vi "New VI.vi"(8 "error in":errorcluster) -> (0 "error out":errorcluster, 3 "VI Refnum":refnum<vi>)   [LabVIEW 2026, in "G-AI Core.lvlib"]
doc: "Creates a new VI and returns it's reference. It's a simple wrapper around the New VI VI-Scripting function. Use this over the original function, since it keeps the VI reference alive even if the tools execution has finished.\n\n_____\nCreated using DQMH Framework: Event Scripter 7.1.2.1547."
uses:
  G-AI Core.lvlib
  New VI Argument--cluster.ctl
  New VI (Reply Payload)--cluster.ctl
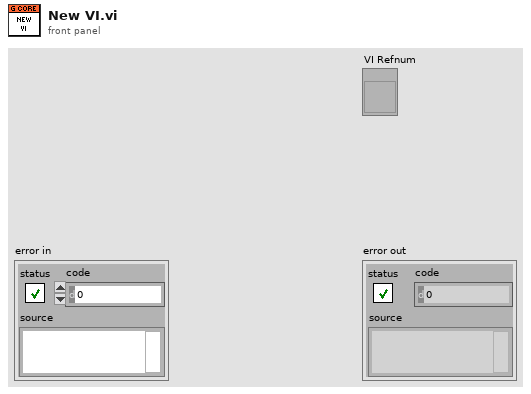
[diagram p1: front panel]
types:
  T1 = typedef "G-AI Core.lvlib/New VI Argument--cluster.ctl" = cluster{"Wait Notifier":refnum<notifier>, "wait for reply":bool}
  T2 = typedef "G-AI Core.lvlib/Request Events--cluster.ctl" = cluster{"Stop Module":refnum<user-event>, "Show Panel":refnum<user-event>, "Hide Panel":refnum<user-event>, "Get Module Execution Status":refnum<user-event>, "Show Diagram":refnum<user-event>, "Store Reference":refnum<user-event>, "Get Reference":refnum<user-event>, "New VI":refnum<user-event>, "Open VI Reference":refnum<user-event>}
  T3 = typedef "G-AI Core.lvlib/New VI (Reply Payload)--cluster.ctl" = cluster{"VI Refnum":refnum<vi>, "error":errorcluster}
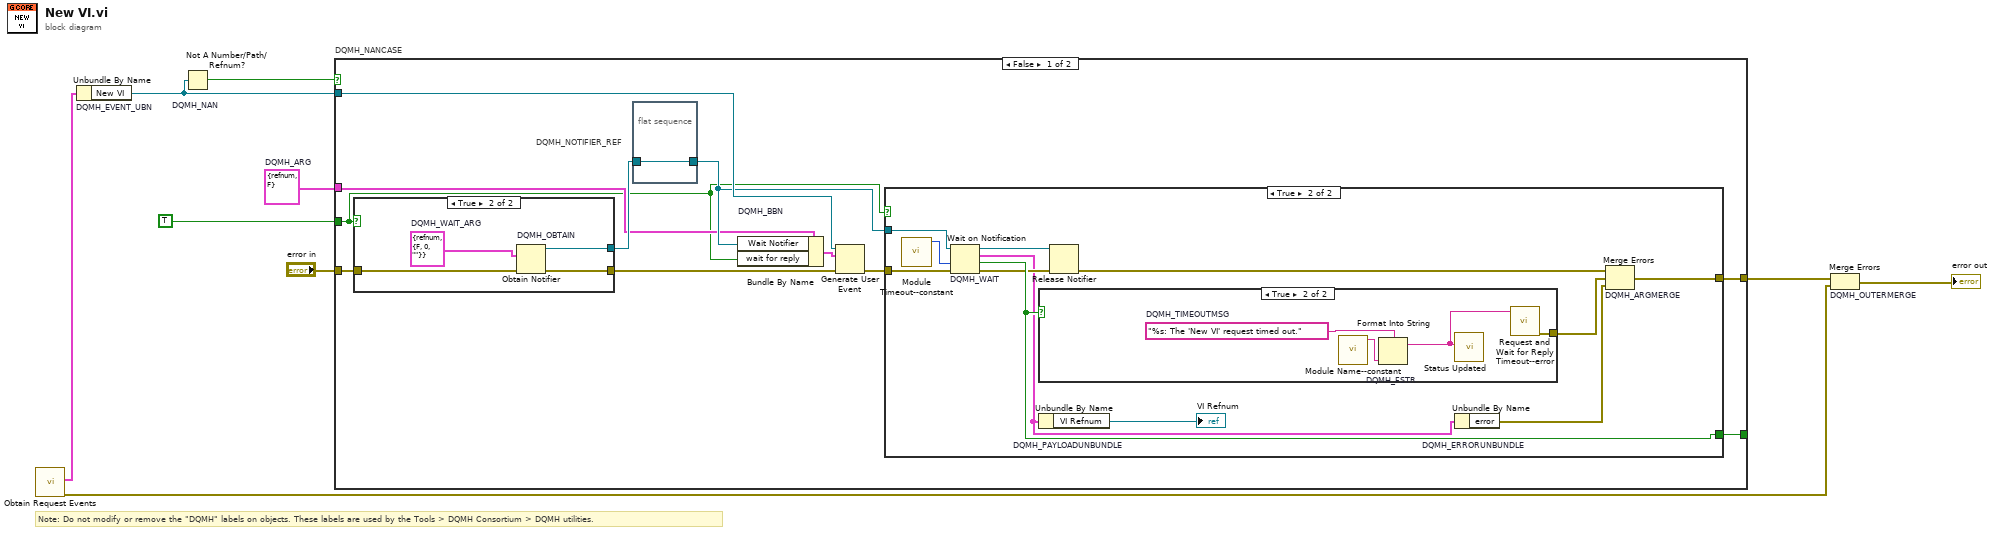
[diagram p0: block diagram]
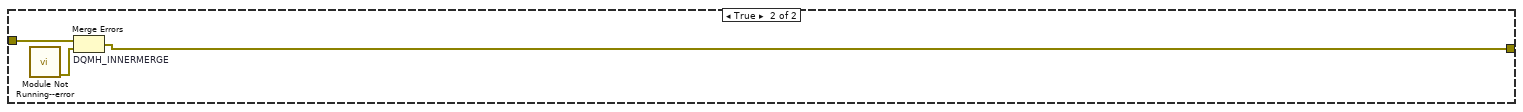
[diagram p5: hidden frame]
diagram:
  w4 = T1 {"Wait Notifier"=refnum, "wait for reply"=FALSE}  # DQMH_ARG
  # "Note: Do not modify or remove the \"DQMH\" labels on objects. These labels are used by the Tools > DQMH Consortium > DQMH utilities."
  n1 = call "Obtain Request Events.vi"() -> ("error out"=w2:errorcluster, "G-AI Core Request Events"=w1:T2)  [unwired: 10 in]
  n2 = Unbundle By Name "DQMH_EVENT_UBN"(w1) -> ("New VI"=w7:refnum<user-event>)
  n3 = Not A Number/Path/Refnum? "DQMH_NAN"(number/path/refnum=w7) -> (NaN/Path/Refnum?=w6:bool)
  n4 = case "DQMH_NANCASE" shown="False" w6 {
    tunnel: "error in" -> [w20 w46]
    tunnel: w7 -> [w18 _]
    tunnel: [w15 w45] -> w5
    tunnel: [w16 _] -> _
    tunnel: w4 -> [w11 _]
    tunnel: TRUE ("wait for reply (T)") -> [w10 _]
    frame False {
      n5 = case shown="True" w10 {
        tunnel: w20 -> [w39 w43]
        tunnel: [w39 w42] -> w17
        tunnel: [_ w40] -> w13
        frame False {
        }
        frame True {
          w41 = T3 {"VI Refnum"=refnum, "error"={"status"=FALSE, "code"=0, "source"=""}}  # DQMH_WAIT_ARG
          n6 = Obtain Notifier "DQMH_OBTAIN"(notification data type=w41, error in (no error)=w43) -> (notifier out=w40:refnum<notifier>, error out=w42:errorcluster)  [unwired: 2 in, 1 out]
        }
      }
      n7 = flat-sequence "DQMH_NOTIFIER_REF" {
        tunnel: w13 -> [w21]
        tunnel: [w21] -> w12
        frame #0 {
        }
      }
      n8 = Bundle By Name "DQMH_BBN"(cluster=w11, "Wait Notifier"=w12, "wait for reply"=w10) -> (w14:T1)
      n9 = Generate User Event(user event=w18, event data cluster=w14, error in=w17) -> (error out=w19:errorcluster)  [unwired: 1 in, 1 out]
      n10 = case shown="True" w10 {
        tunnel: w19 -> [w22 w34]
        tunnel: w12 -> [_ w33]
        tunnel: [_ w31] -> w16
        tunnel: [w22 w30] -> w15
        frame False {
        }
        frame True {
          n11 = call "Module Timeout--constant.vi"() -> ("Module Timeout"=w24:i32)  [unwired: 11 in]
          n12 = Wait on Notification "DQMH_WAIT"(notifier=w33, timeout in ms (-1)=w24, error in (no error)=w34) -> (notifier out=w32:refnum<notifier>, notification=w25:T3, timed out?=w31:bool, error out=w29:errorcluster)  [unwired: 1 in]
          n13 = case shown="True" w31 {
            tunnel: [_ w36] -> w26
            frame False {
            }
            frame True {
              w38 = "%s: The 'New VI' request timed out."  # DQMH_TIMEOUTMSG
              n14 = call "Module Name--constant.vi"() -> ("Module Name"=w35:string)  [unwired: 11 in]
              n15 = Format Into String "DQMH_FSTR"(format string=w38, w35) -> (resulting string=w37:string)  [unwired: 2 in, 1 out]
              n16 = call "Status Updated.vi"("Status"=w37) -> ()  [unwired: 10 in, 1 out]
              n17 = call "Request and Wait for Reply Timeout--error.vi"("Error Message"=w37) -> ("error out"=w36:errorcluster)  [unwired: 10 in]
            }
          }
          n18 = Unbundle By Name "DQMH_PAYLOADUNBUNDLE"(w25) -> ("VI Refnum"=→"VI Refnum":refnum<vi>)
          n19 = Release Notifier(notifier=w32, error in (no error)=w29) -> (error out=w28:errorcluster)  [unwired: 1 in, 2 out]
          n20 = Unbundle By Name "DQMH_ERRORUNBUNDLE"(w25) -> ("error"=w27:errorcluster)
          n21 = Merge Errors "DQMH_ARGMERGE"(w28, w26, w27) -> (w30:errorcluster)
        }
      }
    }
    frame True {
      n22 = call "Module Not Running--error.vi"() -> ("error out"=w44:errorcluster)  [unwired: 11 in]
      n23 = Merge Errors "DQMH_INNERMERGE"(w46, w44) -> (w45:errorcluster)
    }
  }
  n24 = Merge Errors "DQMH_OUTERMERGE"(w5, w2) -> (→"error out":errorcluster)
